vi "Initialize.vi"(6 "Timeout [ms]":u32=10000, 7 "Serial Configuration":T1={"Baud Rate"=9600, "Parity"=0, "Data Bits"=8, "Stop Bits"=20, "Flow Control"=0} {"Flow Control" items=["None", "XON/XOFF", "RTS/CTS", "XON/XOFF & RTS/CTS", "DTR/DSR", "XON/XOFF & DTR/DSR"]; "Stop Bits" items=["1.0"=10, "1.5"=15, "2.0"=20]; "Data Bits" items=["7"=7, "8"=8]; "Parity" items=["None", "Odd", "Even", "Mark", "Space"]; "Baud Rate" items=["300"=300, "600"=600, "1200"=1200, "2400"=2400, "4800"=4800, "9600"=9600, "19200"=19200]}, 8 "error in (no error)":errorcluster, 10 "ID Query (True)":bool, 11 "VISA resource name":refnum<visa-resource-name>) -> (0 "error out":errorcluster, 3 "VISA resource name out":refnum<visa-resource-name>)   [LabVIEW 2017, in "TCxxxx.lvlib"]
doc: "Establishes communication with the instrument and optionally performs an instrument identification query and/or an instrument reset. It also places the instrument in a default state needed for other instrument driver operations. Therefore, call this VI before calling other instrument driver VIs for this instrument. Generally, you need to call the Initialize VI only once at the beginning of an application."
uses:
  TCxxxx.lvlib
  Controls/Adresse.ctl
panel:
  out "Firmware":u16
  # "(c) 2016 - Tameq Schweiz GmbH."
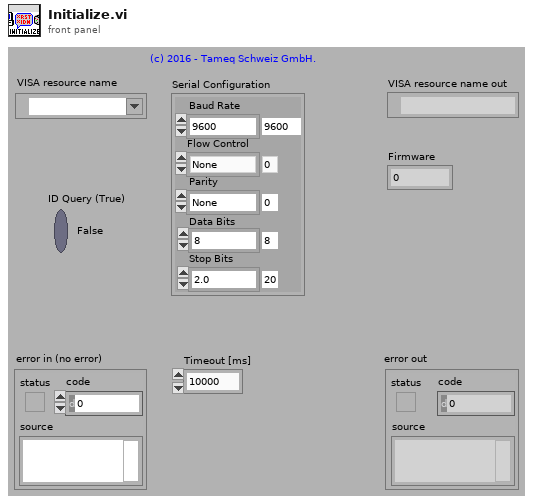
[diagram p1: front panel]
types:
  T1 = cluster{"Baud Rate":u32, "Parity":u16, "Data Bits":u16, "Stop Bits":u16, "Flow Control":u16}
  T2 = typedef "Adresse.ctl" = enum16{"A", "B", "C", "D", "E", "F", "G", "H", "I", "J", "K", "L", "M", "N", "O", "P", "Q", "R", "S", "T", "U", "V", "W", "X", "Y", "Z"}
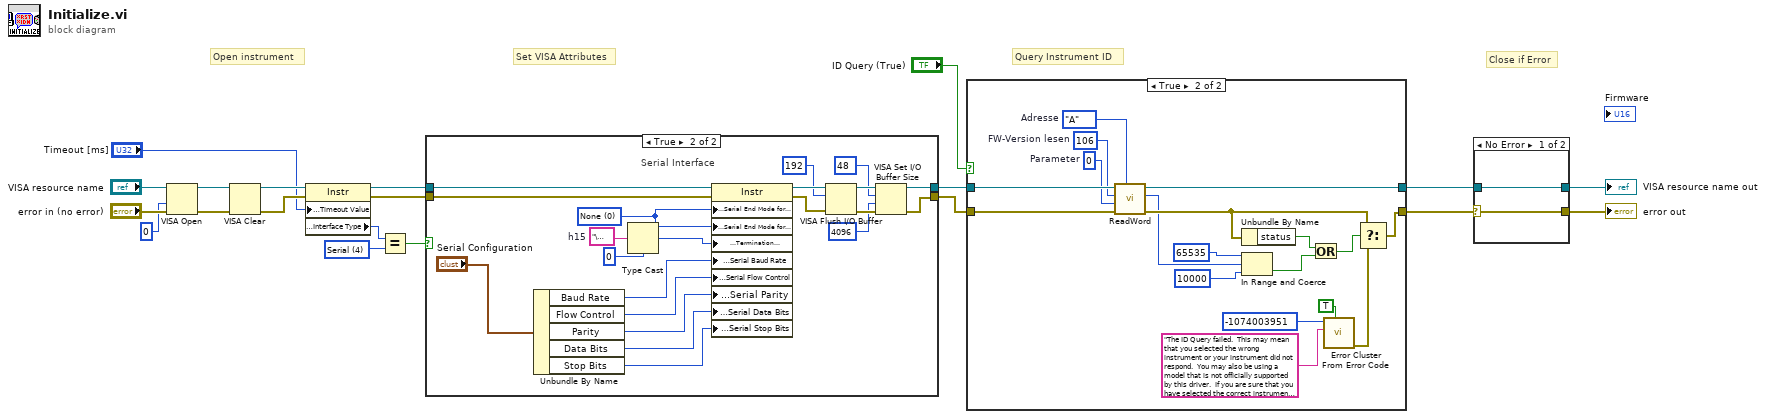
[diagram p0: block diagram]
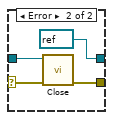
[diagram p3: hidden frame]
diagram:
  w11 = u16 4 items=["GPIB"=1, "VXI"=2, "GPIB-VXI"=3, "Serial"=4, "PXI"=5, "TCPIP"=6, "USB"=7] ("Interface Information:Interface Type")
  # "Set VISA Attributes"
  # "Close if Error"
  # "Query Instrument ID"
  # "Open instrument"
  n1 = VISA Open(access mode=u32 0, error in (no error)="error in (no error)", VISA resource name="VISA resource name") -> (VISA resource name=w9:refnum<visa-resource-name>, error out=w8:errorcluster)  [unwired: 2 in]
  n2 = VISA Clear(VISA resource name=w9, error in (no error)=w8) -> (VISA resource name out=w7:refnum<visa-resource-name>, error out=w6:errorcluster)
  n3 = property class="Instr"(reference=w7, error in=w6, "General Settings:Timeout Value"="Timeout [ms]") -> (reference out=w14:refnum<visa-resource-name>, error out=w13:errorcluster, "Interface Information:Interface Type"=w17:u16)
  n4 = Equal?(x=w17, y=w11) -> (x = y?=w12:bool)
  n5 = case shown="True" w12 {
    tunnel: [w21 w40] -> w16
    tunnel: [w22 w37] -> w15
    tunnel: w14 -> [w21 w42]
    tunnel: w13 -> [w22 w43]
    frame False {
      # "EDIT: Remove interfaces not\nsupported by your instrument."
      # "GPIB, TCP/IP, and USB Interface"
    }
    frame True {
      w23 = "\u0015"  # h15
      w31 = u16 0 items=["None", "LastBit", "TermChar"] ("Serial Settings:Serial End Mode for Reads")
      # "Serial Interface"
      n6 = Unbundle By Name("Serial Configuration") -> ("Baud Rate"=w29:u32, "Flow Control"=w25:u16, "Parity"=w27:u16, "Data Bits"=w28:u16, "Stop Bits"=w24:u16)
      n7 = Type Cast(type=u8 0, x=w23) -> (*(type *) &x=w30:u8)
      n8 = property class="Instr"(reference=w42, error in=w43, "Serial Settings:Serial End Mode for Reads"=w31, "Serial Settings:Serial End Mode for Writes"=w31, "Message Based Settings:Termination Character"=w30, "Serial Settings:Serial Baud Rate"=w29, "Serial Settings:Serial Flow Control"=w25, "Serial Settings:Serial Parity"=w27, "Serial Settings:Serial Data Bits"=w28, "Serial Settings:Serial Stop Bits"=w24) -> (reference out=w36:refnum<visa-resource-name>, error out=w39:errorcluster)
      n9 = VISA Flush I/O Buffer(VISA resource name=w36, mask (16)=u16 192, error in (no error)=w39) -> (VISA resource name out=w41:refnum<visa-resource-name>, error out=w38:errorcluster)
      n10 = VISA Set I/O Buffer Size(VISA resource name=w41, mask (16)=u16 48, size (4096)=u32 4096 ("size (0)"), error in (no error)=w38) -> (VISA resource name out=w40:refnum<visa-resource-name>, error out=w37:errorcluster)
    }
  }
  n11 = case shown="True" "ID Query (True)" {
    tunnel: [w44 w63] -> w2
    tunnel: [w45 w55] -> w3
    tunnel: w16 -> [w45 w56]
    tunnel: w15 -> [w44 w54]
    frame False {
    }
    frame True {
      w50 = u16 0  # Parameter
      w51 = Adresse."A"  # Adresse
      w52 = u16 106  # FW-Version lesen
      n12 = call "ReadWord.vi"("Adresse"=w51, "error in (no error)"=w54, "Parameter [0 ... 65535]"=w50, "Befehl [0 ... 65535]"=w52, "VISA resource name"=w56) -> ("error out"=w53:errorcluster, "Regler Rückgabewert [0 ... 65535]"=w47:u16, "VISA resource name out"=w55:refnum<visa-resource-name>)  [unwired: 3 in, 1 out]
      n13 = Unbundle By Name(w53) -> ("status"=w58:bool)
      n14 = In Range and Coerce(upper limit=65535, x=w47, lower limit=10000) -> (In Range?=w46:bool)  [unwired: 1 out]
      n15 = Or(x=w58, y=w46) -> (x .or. y?=w57:bool)
      n16 = call <vilib>:"Error Cluster From Error Code.vi"("show call chain? (False)"=TRUE, "error message (\"\")"="The ID Query failed.  This may mean that you selected the wrong instrument or your instrument did not respond.  You may also be using a model that is not officially supported by this driver.  If you are sure that you have selected the correct instrument and it is responding, try disabling the ID Query." ("Source (VI Name)"), "error code (0)"=-1074003951 ("Code")) -> ("error out"=w62:errorcluster)  [unwired: 6 in]
      n17 = Select(t=w53, s=w57, f=w62) -> (s? t:f=w63:errorcluster)
    }
  }
  n18 = case shown="No Error" w2 {
    selector: w2 -> [w64 w67]
    tunnel: w3 -> [w65 w68]
    tunnel: [w65 refnum<visa-resource-name> refnum ("VISA resource name out")] -> w5
    tunnel: [w64 w69] -> w4
    frame No Error {
    }
    frame Error {
      n19 = call "Close.vi"("error in (no error)"=w67, "VISA resource name"=w68) -> ("error out"=w69:errorcluster)  [unwired: 9 in]
    }
  }
  "VISA resource name out" <- w5
  "error out" <- w4
